vi "Define Abstractly.vi"(10 "Relation Definition":T1, 11 "Relation in":refnum<class "Relation.lvclass">) -> (3 "Relation out":refnum<class "Relation.lvclass">)   [LabVIEW 2020, in "Conditum.lvlib" / "Columns.lvlib" / "Relation.lvclass"]
uses:
  Relation.lvclass
  Relation.lvclass/Relation.ctl
  Type/Definition.ctl
  Type/Type.lvclass
  Relation Mapping.ctl
  Conditum.lvlib
  Relation Info.ctl
  Relation Definition.ctl
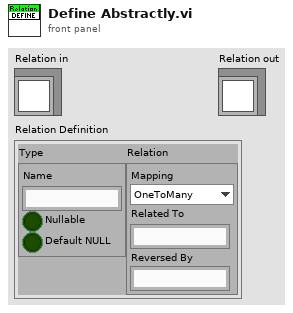
[diagram p1: front panel]
types:
  T1 = typedef "Conditum.lvlib/Columns.lvlib/Relation.lvclass/Relation Definition.ctl" = cluster{"Type":T2, "Relation":T3}
  T2 = typedef "Conditum.lvlib/Columns.lvlib/Type.lvclass/Definition.ctl" = cluster{"Name":string, "Nullable":bool, "Default NULL":bool}
  T3 = typedef "Conditum.lvlib/Relation Info.ctl" = cluster{"Mapping":T4, "Related To":string, "Reversed By":string}
  T4 = typedef "Conditum.lvlib/Relation Mapping.ctl" = enum16{"OneToMany", "ManyToOne", "ManyToMany", "OneToOne"}
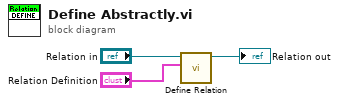
[diagram p0: block diagram]
diagram:
  n1 = call "Define Relation.vi"("Relation Definition"="Relation Definition", "Relation in"="Relation in") -> ("Relation out"=→"Relation out":refnum<class "Relation.lvclass">)  [unwired: 9 in]
